vi "WPI_IMU_ADIS16448_WriteCommand.vi"(8 "error in (no error)":errorcluster, 9 "Data":u16=2049, 11 "SPIDevRef in":T1) -> (0 "error out":errorcluster, 3 "SPIDevRef out":T1)   [LabVIEW 2015, in "Apple Pi Gyro Library.lvlib" / "FRC_ADIS16448_IMU.lvlib"]
uses:
  FRC_ADIS16448_IMU.lvlib
  <vilib>/Rock Robotics/WPI/SPI/WPI_SPIDevRef.ctl
  <vilib>/Rock Robotics/SystemInterfaces/spilib/spi_bus.ctl
  WPI_IMU_ADIS16448_Registers.ctl
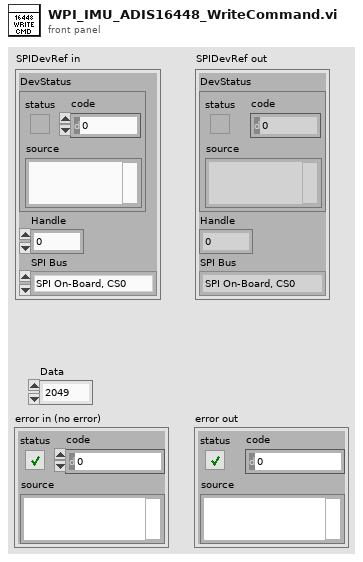
[diagram p1: front panel]
types:
  T1 = typedef "WPI_SPIDevRef.ctl" = cluster{"DevStatus":errorcluster, "Handle":i32, "SPI Bus":T2}
  T2 = typedef "spi_bus.ctl" = enum16{"SPI On-Board, CS0", "SPI On-Board, CS1", "SPI On-Board, CS2", "SPI On-Board, CS3", "SPI MXP", "Invalid"}
  T3 = typedef "Apple Pi Gyro Library.lvlib/FRC_ADIS16448_IMU.lvlib/WPI_IMU_ADIS16448_Registers.ctl" = u8
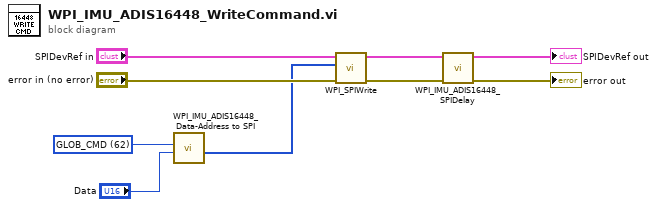
[diagram p0: block diagram]
diagram:
  w9 = T3 62 items=["GLOB_CMD"=62, "SEQ_CNT"=58, "SMPL_PRD"=54, "SENS_AVG"=56, "MSC_CTRL"=52, "ERROR_FLAGS"=60, "TEMP"=44, "BARO"=40, "Z_MAG"=36, "Y_MAG"=32, "X_MAG"=28, "Z_ACCEL"=24, "Y_ACCEL"=20, "X_ACCEL"=16, "Z_GYRO"=12, "Y_GYRO"=8, "X_GYRO"=4, "PROD_ID"=86, "LOT_ID2"=84, "LOT_ID1"=82, "SERIAL_NUM"=88] ("ADIS16448 Register")
  n1 = call "WPI_IMU_ADIS16448_Data-Address to SPI.vi"("Data"="Data", "Address"=w9) -> ("Low Word"=w5:u8[])  [unwired: 8 in, 1 out]
  n2 = call <vilib>:"WPI_SPIWrite.vi"("error in (no error)"="error in (no error)", "Data To Send"=w5, "SPIDevRef"="SPIDevRef in") -> ("error out"=w3:errorcluster, "SPIDevRef"=w4:T1)  [unwired: 7 out]
  n3 = call "WPI_IMU_ADIS16448_SPIDelay.vi"("error in"=w3, "SPIDevRef in"=w4) -> ("error out"=→"error out":errorcluster, "SPIDevRef out"=→"SPIDevRef out":T1)  [unwired: 8 in]
